vi "find best origin.vi"(11 "address":string) -> (3 "origin":string)   [LabVIEW 2016, in "websocket client.lvclass"]
uses:
  websocket client.lvclass
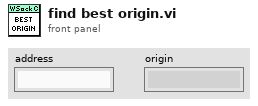
[diagram p1: front panel]
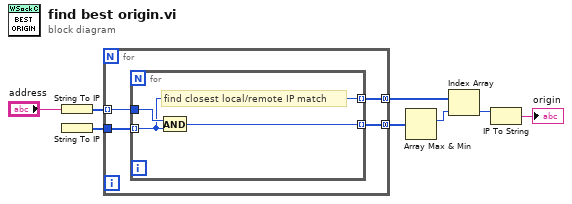
[diagram p0: block diagram]
diagram:
  n1 = String To IP(1:"address") -> (0:w3:u32[])
  n2 = String To IP() -> (0:w4:u32[])  [unwired: 1 in]
  n3 = for {
    tunnel: w3 -> [w11] mode=indexing
    tunnel: w4 -> [w12]
    tunnel: [w10] -> w5 mode=concatenating
    tunnel: [w9] -> w6 mode=concatenating
    n4 = for {
      tunnel: w12 -> [w13] mode=indexing
      tunnel: w11 -> [w15]
      tunnel: [w14] -> w10 mode=indexing
      tunnel: [w13] -> w9 mode=indexing
      # "find closest local/remote IP match"
      n5 = And(x=w15, y=w13) -> (x .and. y?=w14:u32)
    }
  }
  n6 = Array Max & Min(array=w5) -> (max index (indices)=w7:i32)  [unwired: 3 out]
  n7 = Index Array(array=w6, index=w7) -> (element=w8:u32)
  n8 = IP To String(2:w8) -> (0:→"origin":string)  [unwired: 1 in]
